vi "GT Follow Data.vi"(5 "fifo":i16, 6 "type":i16, 7 "slaveSegment":dbl, 8 "error in (no error)":errorcluster caption="错误输入（无错误）", 9 "masterSegment":i32, 10 "profile":i16, 11 "cardNum":i16) -> (0 "error out":errorcluster caption="错误输出", 3 "function return":i16)   [LabVIEW 2014, in "gts.lvlib"]
doc: "GT_API GT_FollowData(short cardNum,short profile,long masterSegment,double slaveSegment,short type=FOLLOW_SEGMENT_NORMAL,short fifo=0);"
uses:
  gts.lvlib
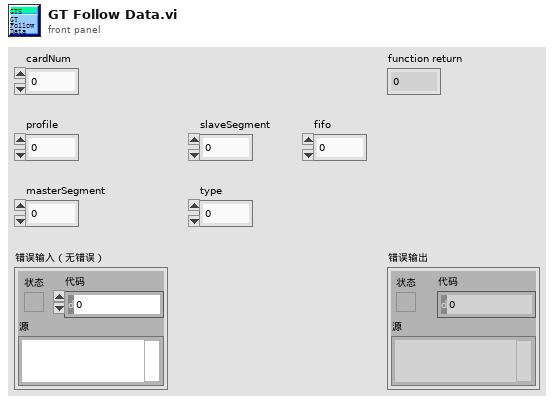
[diagram p1: front panel]
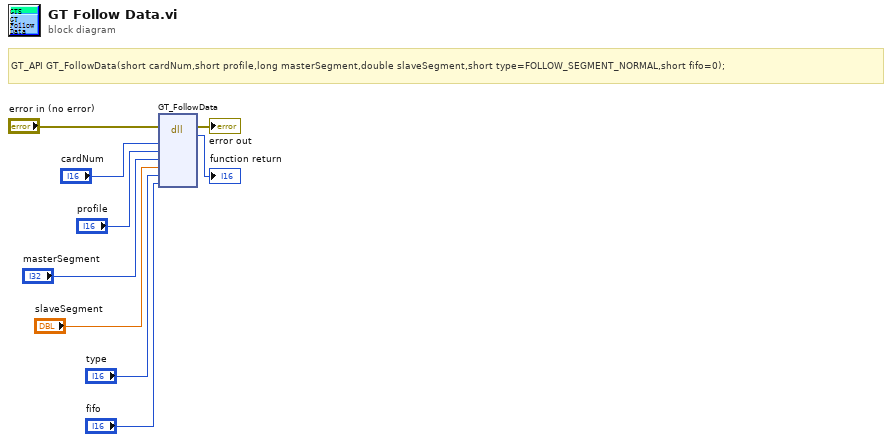
[diagram p0: block diagram]
diagram:
  # "GT_API GT_FollowData(short cardNum,short profile,long masterSegment,double slaveSegment,short type=FOLLOW_SEGMENT_NORMAL,short fifo=0);"
  n1 = dll-call lib="PTH2habs D固高科技资料GTS控制卡GTS卡18年上半年资料dllVC32bit\nmulti_cardgts.*" fn="GT_FollowData"(error in="error in (no error)", "cardNum"="cardNum", "profile"="profile", "masterSegment"="masterSegment", "slaveSegment"="slaveSegment", "type"="type", "fifo"="fifo") -> (error out=→"error out":errorcluster, →"function return":i16)  [unwired: 8 in, 1 out]
